vi "Check DAQ Status.vi"(0 "errIN":errorcluster, 1 "TL Calling Location":string, 3 "Task ID":u32 format="%.0x") -> (2 "error out":errorcluster, 5 "Armed?":bool)   [LabVIEW 2015]
doc: "DESCRIPTION:\nThis VI counts rising edges, using an NI-TIO based device (e.g.: 6602). The counter increments its event count everytime a pulse comes into its source input. The counters only increments between the rising edge of the aux line and the rising edge of the gate. The current value of the counter is read when the counter is finished or an error occurs. \n\n\n\nINSTRUCTIONS:\n1. Enter the device and counter you want use.\n2. Optional controls are located on the left side of the front panel. You will have to use your scroll bar to reach these. \n3. Connect your signals as described below in I/O CONNECTIONS.\n4. Run the VI.\n\n\nKEY PARAMETERS:\nCounter Group Config.vi: task type = two edge separation measurement\nCounter Source (NI-TIO).vi: Source Specification\nCounter Gate (NI-TIO).vi: Gate Specification\nCounter Aux Line (NI-TIO): Aux Line Specification\nCounter Get Attribute.vi: armed, TC Reached, count\nCounter Control.vi: Program, Reset\n\n\n\nI/O CONNECTIONS:\nConnect the start signal to the aux line input of the selected counter. Connect the stop signal to the gate input of the selected counter. \nIf you selected the Source Selection to be \"PFI line\", connect your event count base signal to the PFI line indicated by \"Source PFI line number used\". (If you selected \"Internal Timebase\", no source connection is necessary.)\n\nNOTE: For actual I/O pin numbers, please refer to your hardware user manual.\n\n\n\nDAQ VIs USED:\nCounter Group Config.vi\nCounter Source (NI-TIO).vi\nCounter Gate (NI-TIO).vi\nCounter Aux Line (NI-TIO)\nCounter Get Attribute.vi\nCounter Control.vi"
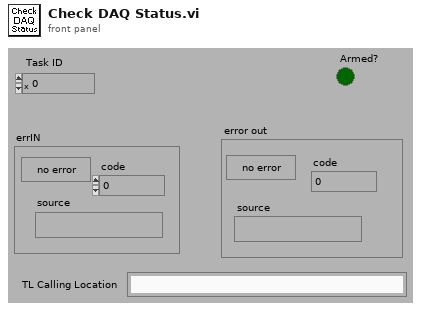
[diagram p1: front panel]
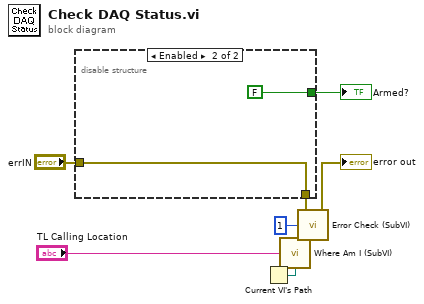
[diagram p0: block diagram]
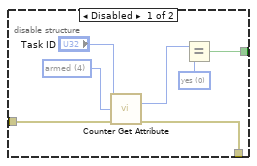
[diagram p2: hidden frame]
diagram:
  n1 = disable-structure shown="Enabled" {
    disable-tunnel: [w11 FALSE ("Armed?")] -> w8
    disable-tunnel: "errIN" -> [w10 w16]
    disable-tunnel: [w9 w16] -> w2
    frame Disabled {
      w14 = u32 0 items=["yes", "no", "high", "low"] ("attribute value type")
      w15 = u32 4 items=["count", "saved count", "count available", "available points", "armed", "TC reached", "done", "output state", "read mark", "write mark", "internal max timebase", "max prescale", "read mark high snapshot", "read mark low snapshot", "write mark high snapshot", "write mark low snapshot", "backlog high snapshot", "backlog low snapshot", "armed snapshot"] ("attribute ID")
      n2 = call <vilib>:"Counter Get Attribute.vi"("task ID"="Task ID", "attribute ID"=w15, "error in (no error)"=w10) -> ("attribute value type"=w13:u32, "error out"=w9:errorcluster)  [unwired: 11 out]
      n3 = Equal?(x=w13, y=w14) -> (x = y?=w11:bool)
    }
    frame Enabled {
    }
  }
  "Armed?" <- w8
  n4 = Current VI's Path() -> (path=w6:path)
  n5 = call "Where Am I (SubVI).vi"("TL Calling Location"="TL Calling Location", "Call VI path"=w6) -> ("I'm here"=w5:string)
  n6 = call "Error Check (SubVI).vi"("calling VI"=w5, "tag #"=1 ("code locator tag #"), "error IN"=w2) -> ("error OUT"=→"error out":errorcluster)  [unwired: 2 out]
